vi "Acquisition Message Loop.vi"(8 "error in (no error)":errorcluster, 9 "Data Queue":refnum<queue>, 10 "Data Notifier":refnum<notifier>, 11 "Message Queues":T1) -> (0 "error out":errorcluster)   [LabVIEW 2018, in "Acquisition.lvlib"]
doc: "Message loop for handling messages pertaining to the acquisition of data from the hardware."
uses:
  Acquisition.lvlib
  support/Message Queue/All Message Queues.ctl
  support/Message Queue/Message Cluster.ctl
  Hardware Configuration.ctl
  Acquisition State.ctl
  <vilib>/Platform/TimedLoop/XDataNode/timing_clust.ctl
  <vilib>/Platform/TimedLoop/XDataNode/nitl_modes.ctl
  <vilib>/Platform/TimedLoop/XDataNode/wakeup.ctl
  support/Message Queue/Enqueue Message (Single).vi
  <vilib>/Utility/error.llb/Error Cluster From Error Code.vi
  <vilib>/platform/TimedLoop/XDataNode/XDataNode.xnode
  <vilib>/ErrorRing/Error Ring.xnode
  support/Message Queue/Message Queue.lvlib
  <vilib>/Platform/TimedLoop/XDataNode/XDNodeRunTimeDep.lvlib
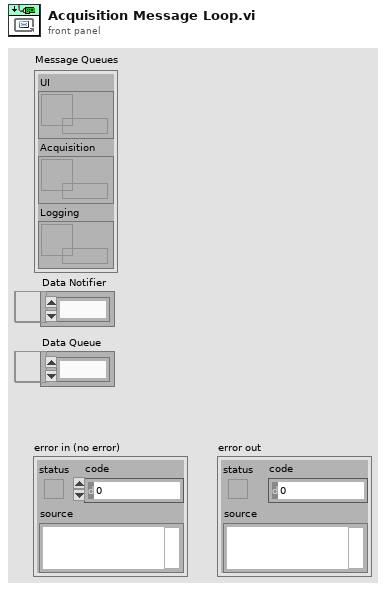
[diagram p1: front panel]
types:
  T1 = typedef "Message Queue.lvlib/All Message Queues.ctl" = cluster{"UI":refnum<queue>, "Acquisition":refnum<queue>, "Logging":refnum<queue>}
  T2 = typedef "Acquisition.lvlib/Hardware Configuration.ctl" = cluster{"DAQmx Channel 1":tag, "DAQmx Channel 2":tag, "DAQmx Channel 3":tag, "DAQmx AI Task":refnum<k21>, "Channel 1 Name":string, "Channel 2 Name":string, "Channel 3 Name":string, "Sample time":u32, "Samples per second":dbl, "Sample mode":u16, "Samples per channel":i32, "Offset Channel 1":dbl, "Offset Channel 2":dbl, "Offset Channel 3":dbl, "Scale Channel 1":dbl, "Scale Channel 2":dbl, "Scale Channel 3":dbl, "DAQmx Counter Channel":tag, "Counter Name":string, "DAQmx Counter Task":refnum<k21>}
  T3 = typedef "XDNodeRunTimeDep.lvlib/timing_clust.ctl" = cluster{"Expected End [f-1]":u64, "Actual End [f-1]":u64, "Finished Late? [f-1]":bool, "Expected End [i-1]":u64, "Actual End [i-1]":u64, "Finished Late? [i-1]":bool, "Expected Start [i]":u64, "Actual Start [i]":u64, "Expected Start [f]":u64, "Actual Start [f]":u64, "Source Name":string, "Structure Name":string, "Period":i64, "Deadline":i64, "Offset":i64, "Start":i64, "Priority":i32, "Timeout":i32, "Mode":T4, "Wakeup Reason":T5, "Error":errorcluster, "Source Type":string, "Secondary Source Type":string, "Global End Time":u64, "Global Start Time":u64, "Frame Duration":u64, "Iteration Duration":u64, "Assigned CPU":i32, "I/O Scan Engine Mode":u32}
  T4 = typedef "XDNodeRunTimeDep.lvlib/nitl_modes.ctl" = enum32{"No Change", "Process missed periods, maintain original phase", "Discard missed periods, maintain original phase", "Process missed periods, ignore original phase", "Discard missed periods, ignore original phase"}
  T5 = typedef "XDNodeRunTimeDep.lvlib/wakeup.ctl" = enum32{"Normal", "Aborted", "Asynchronous wakeup", "Timing source error", "Timed loop error", "Timeout"}
  T6 = typedef "Acquisition.lvlib/Acquisition State.ctl" = enum16{"Idle", "Acquiring"}
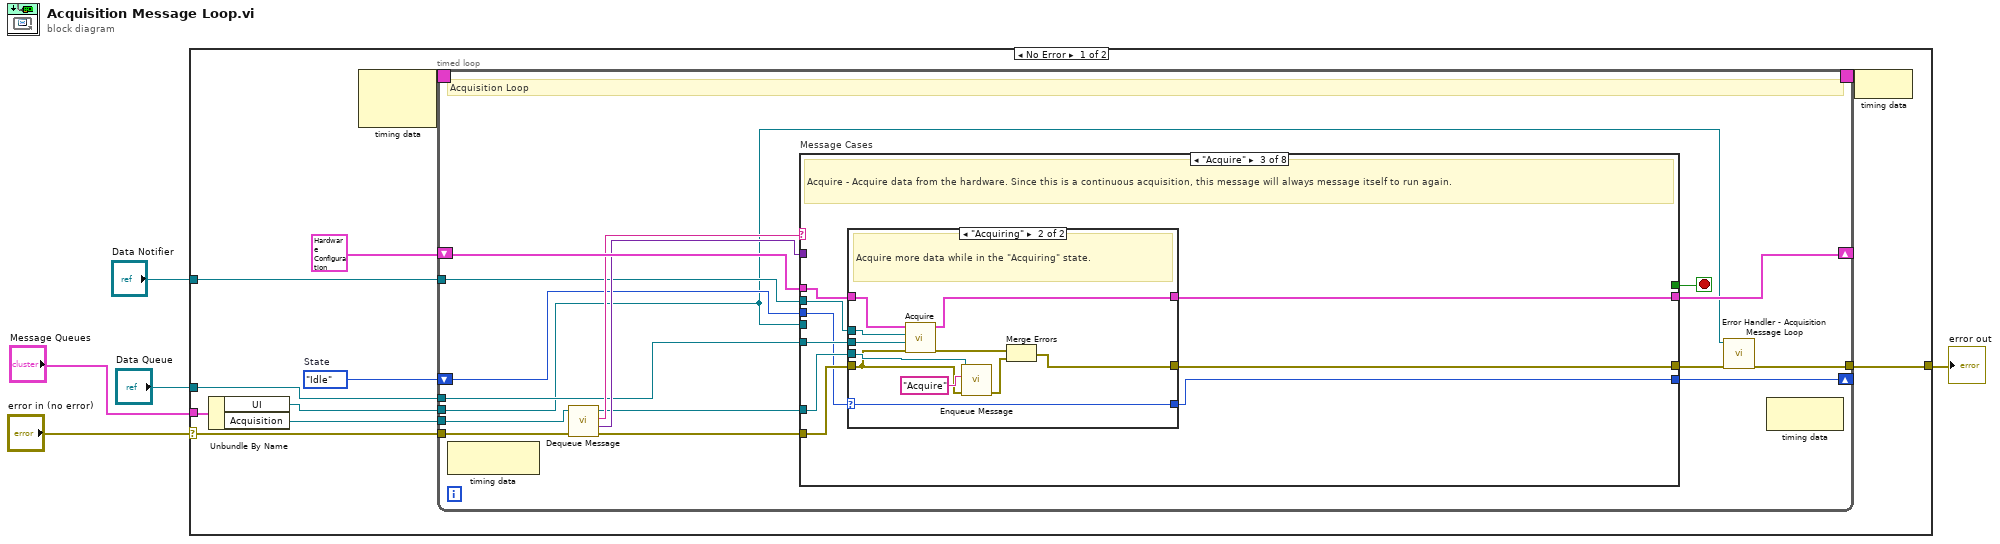
[diagram p0: block diagram]
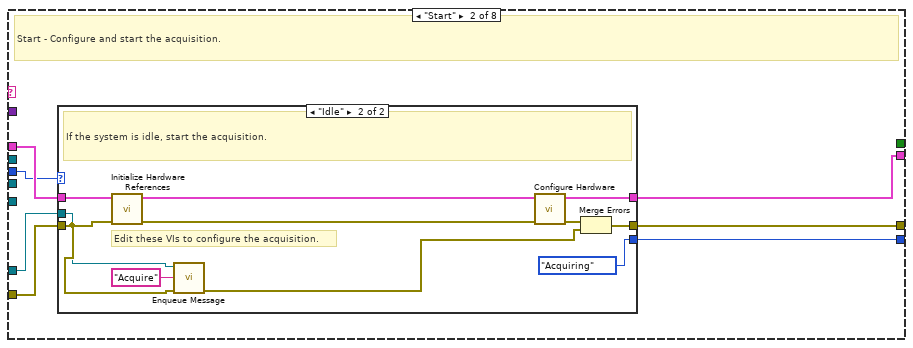
[diagram p3: hidden frame]
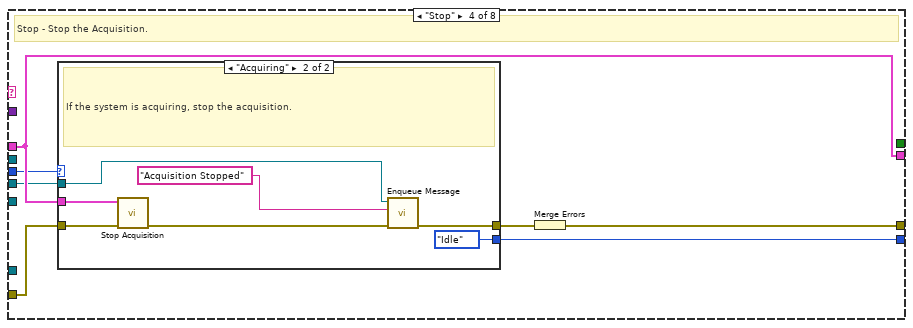
[diagram p6: hidden frame]
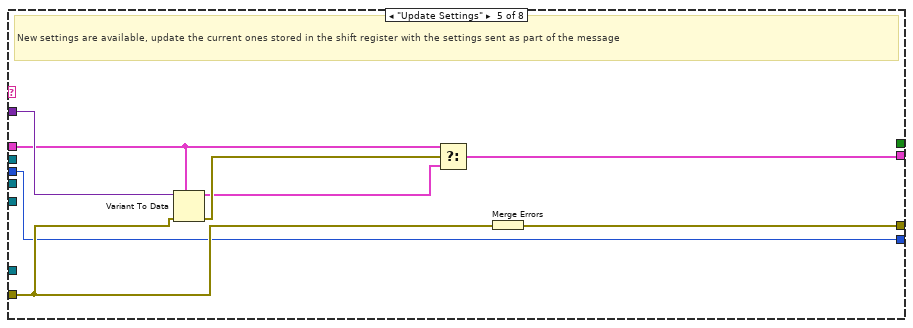
[diagram p8: hidden frame]
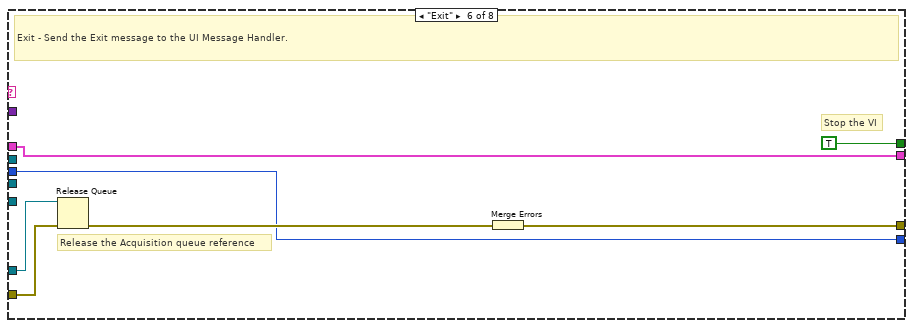
[diagram p9: hidden frame]
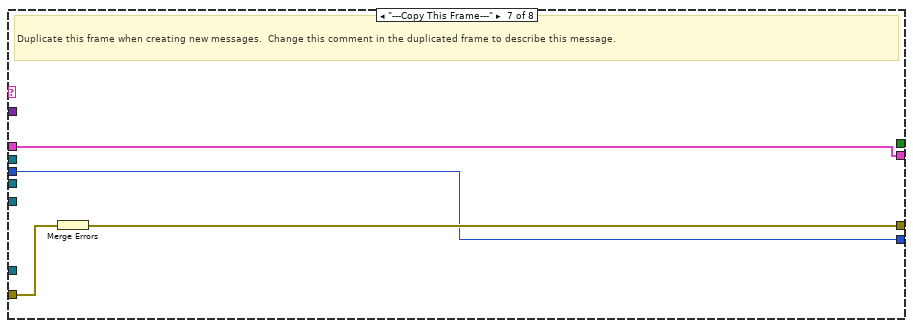
[diagram p10: hidden frame]
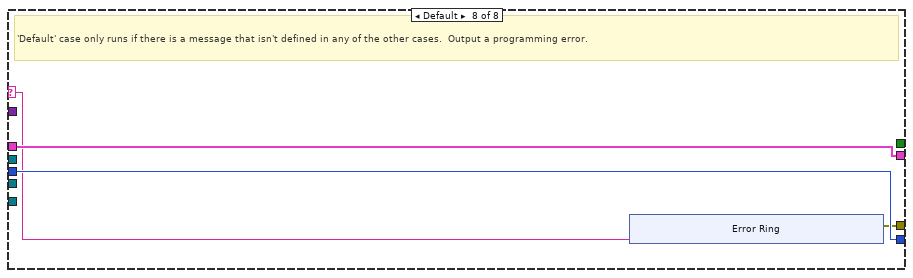
[diagram p11: hidden frame]
diagram:
  n1 = case shown="No Error" "error in (no error)" {
    selector: "error in (no error)" -> [w13 w130]
    tunnel: "Message Queues" -> [w16 _]
    tunnel: [w14 w130] -> w4
    tunnel: "Data Notifier" -> [w11 _]
    tunnel: "Data Queue" -> [w10 _]
    frame No Error {
      w9 = Acquisition_State."Idle"  # State
      n2 = Unbundle By Name(w16) -> ("UI"=w12:refnum<queue>, "Acquisition"=w15:refnum<queue>)
      n3 = node-c288() -> (w8:T3)  [unwired: 2 in]
      n4 = timed-loop {
        tunnel: w15 -> [w25]
        shift-right: [w31] -> _
        shift-left: T2 {"DAQmx Channel 1"="", "DAQmx Channel 2"="", "DAQmx Channel 3"="", "DAQmx AI Task"="", "Channel 1 Name"="Battery Voltage", "Channel 2 Name"="Battery Current", "Channel 3 Name"="Brake torque", "Sample time"=50, "Samples per second"=1000.0, "Sample mode"=0, "Samples per channel"=0, "Offset Channel 1"=0.0, "Offset Channel 2"=0.0, "Offset Channel 3"=0.0, "Scale Channel 1"=0.0, "Scale Channel 2"=0.0, "Scale Channel 3"=0.0, "DAQmx Counter Channel"="", "Counter Name"="", "DAQmx Counter Task"=""} ("Data Cluster") -> [w32]
        tunnel: w12 -> [w17]
        tunnel: w11 -> [w24]
        tunnel: w10 -> [w23]
        shift-right: [w21] -> _
        shift-left: w9 -> [w22]
        tunnel: w13 -> [w29]
        tunnel: [w20] -> w14
        timing: w8 -> [_]
        timing-out: [_] -> w7
        stop <- w30 stop-if-true
        # "Acquisition Loop"
        n5 = node-c288() -> ()  [unwired: 1 in, 1 out]
        n6 = call "Dequeue Message.vi"("error in (no error)"=w29, "Message Queue"=w25) -> ("error out"=w28:errorcluster, "Message Data"=w26:variant, "Message"=w27:string, "dup Message Queue"=w18:refnum<queue>)  [unwired: 6 in]
        n7 = case "Message Cases" shown="\"Acquire\"" w27 {
          selector: w27 -> [_ _ _ _ _ _ _ w117]
          tunnel: w18 -> [_ w41 w66 _ _ w107 _ _]
          tunnel: w28 -> [w37 w42 w65 w87 w99 w109 w116 _]
          tunnel: [w37 w44 w67 w88 w105 w111 w114 w118] -> w19
          tunnel: w32 -> [w36 w43 w63 w85 w101 w110 w115 w120]
          tunnel: [w36 w40 w64 w85 w100 w110 w115 w120] -> w31
          tunnel: [_ _ _ _ _ TRUE _ _] -> w30
          tunnel: w26 -> [_ _ _ _ w104 _ _ _]
          tunnel: w17 -> [_ _ _ w82 _ _ _ _]
          tunnel: w24 -> [_ _ w62 _ _ _ _ _]
          tunnel: w23 -> [_ _ w61 _ _ _ _ _]
          tunnel: w22 -> [w35 w38 w59 w84 w98 w106 w113 w119]
          tunnel: [w35 w39 w60 w83 w98 w106 w113 w119] -> w21
          frame "Initialize" {
            # "Initialize  - Initialize is currently a no-op.  The hardware initialization takes place in the 'Start' message."
          }
          frame "Start" {
            # "Start - Configure and start the acquisition."
            n8 = case shown="\"Idle\"" w38 {
              selector: w38 -> [w45 _]
              tunnel: [w46 w58] -> w44
              tunnel: w43 -> [w47 w57]
              tunnel: w42 -> [w46 w56]
              tunnel: w41 -> [_ w54]
              tunnel: [w47 w50] -> w40
              tunnel: [w45 Acquisition_State."Acquiring" ("Acquisition State")] -> w39
              frame "Acquiring" {
                # "The system is already acquiring. Ignore the \"Start\" message."
              }
              frame "Idle" {
                # "Edit these VIs to configure the acquisition."
                # "If the system is idle, start the acquisition."
                n9 = call "Initialize Hardware References.vi"("error in (no error)"=w56, "Hardware Resources in"=w57) -> ("error out"=w53:errorcluster, "Hardware Resources out"=w51:T2)  [unwired: 8 in]
                n10 = call-poly "Enqueue Message.vi"("error in (no error)"=w56, "Message"="Acquire", "Message Queue"=w54) -> ("error out"=w55:errorcluster)  [unwired: 7 in, 1 out]
                n11 = call "Configure Hardware.vi"("error in (no error)"=w53, "Hardware Resources in"=w51) -> ("error out"=w52:errorcluster, "Hardware Resources out"=w50:T2)  [unwired: 8 in]
                n12 = Merge Errors(w52, w55) -> (w58:errorcluster)
              }
            }
          }
          frame "Acquire" {
            # "Acquire - Acquire data from the hardware. Since this is a continuous acquisition, this message will always message itself to run again."
            n13 = case shown="\"Acquiring\"" w59 {
              selector: w59 -> [w68 w72]
              tunnel: [w69 w81] -> w67
              tunnel: w66 -> [_ w79]
              tunnel: w65 -> [w69 w71]
              tunnel: [w70 w77] -> w64
              tunnel: w63 -> [w70 w76]
              tunnel: w62 -> [_ w74]
              tunnel: w61 -> [_ w73]
              tunnel: [w68 w72] -> w60
              frame "Idle" {
                # "Ignore \"Acquire\" messages when the acquisition is idle."
              }
              frame "Acquiring" {
                # "Acquire more data while in the \"Acquiring\" state."
                n14 = call "Acquire.vi"("error in (no error)"=w71, "Data Queue"=w73, "Data Notifier"=w74, "Hardware Resources in"=w76) -> ("error out"=w78:errorcluster, "Hardware Resources out"=w77:T2)  [unwired: 6 in]
                n15 = call-poly "Enqueue Message.vi"("error in (no error)"=w71, "Message"="Acquire", "Message Queue"=w79) -> ("error out"=w80:errorcluster)  [unwired: 7 in, 1 out]
                n16 = Merge Errors(w78, w80) -> (w81:errorcluster)
              }
            }
          }
          frame "Stop" {
            # "Stop - Stop the Acquisition."
            n17 = case shown="\"Acquiring\"" w84 {
              selector: w84 -> [w89 _]
              tunnel: w87 -> [w90 w97]
              tunnel: [w90 w93] -> w86
              tunnel: w85 -> [_ w95]
              tunnel: [w89 Acquisition_State."Idle" ("State")] -> w83
              tunnel: w82 -> [_ w92]
              frame "Idle" {
                # "The system is already idle. Ignore the \"Stop\" message."
              }
              frame "Acquiring" {
                # "If the system is acquiring, stop the acquisition."
                n18 = call "Stop Acquisition.vi"("error in (no error)"=w97, "Hardware Resources in"=w95) -> ("error out"=w96:errorcluster)  [unwired: 9 in]
                n19 = call-poly "Enqueue Message.vi"("error in (no error)"=w96, "Message"="Acquisition Stopped", "Message Queue"=w92) -> ("error out"=w93:errorcluster)  [unwired: 7 in, 1 out]
              }
            }
            n20 = Merge Errors(w86) -> (w88:errorcluster)
          }
          frame "Update Settings" {
            # "New settings are available, update the current ones stored in the shift register with the settings sent as part of the message"
            n21 = Variant To Data(error in=w99, type=w101, Variant=w104) -> (data=w102:T2, error out=w103:errorcluster)
            n22 = Select(t=w101, s=w103, f=w102) -> (s? t:f=w100:T2)
            n23 = Merge Errors(w99) -> (w105:errorcluster)
          }
          frame "Exit" {
            # "Release the Acquisition queue reference"
            # "Stop the VI"
            # "Exit - Send the Exit message to the UI Message Handler."
            n24 = Release Queue(queue=w107, error in (no error)=w109) -> (error out=w108:errorcluster)  [unwired: 1 in, 2 out]
            n25 = Merge Errors(w108) -> (w111:errorcluster)
          }
          frame "---Copy This Frame---" {
            # "Duplicate this frame when creating new messages.  Change this comment in the duplicated frame to describe this message."
            n26 = Merge Errors(w116) -> (w114:errorcluster)
          }
          frame Default {
            # "'Default' case only runs if there is a message that isn't defined in any of the other cases.  Output a programming error."
            n27 = xnode "Error Ring"("parameter 0"=w117) -> ("error out"=w118:errorcluster)
          }
        }
        n28 = call "Error Handler - Acquisition Message Loop.vi"("error in (no error)"=w19, "Message Queue"=w17) -> ("dup error in"=w20:errorcluster)  [unwired: 8 in, 1 out]
        n29 = node-c288() -> ()  [unwired: 1 in, 1 out]
      }
      n30 = node-c288(w7) -> ()
    }
    frame Error {
    }
  }
  "error out" <- w4
